vi "FTW-JSON-Object-DeleteElement.vi"(0 "JSON":T1, 5 "Key":string, 11 "error in":errorcluster) -> (4 "JSON out":T1, 6 "Found and Removed?":bool, 15 "error out":errorcluster)   [LabVIEW 2015]
uses:
  core/type/FTW-Type-JSON.ctl
panel:
  # "Inputs"
  # "Outputs"
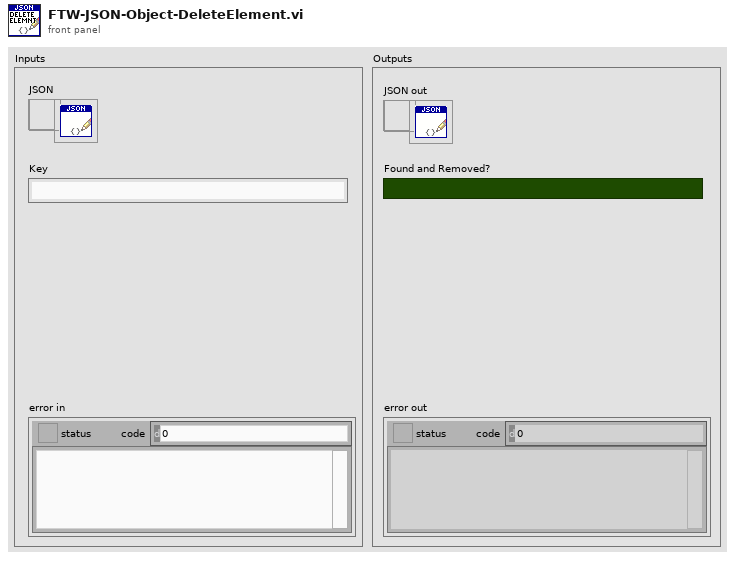
[diagram p1: front panel]
types:
  T1 = typedef "FTW-Type-JSON.ctl" = refnum<data-value>
  T2 = cluster{"FTW-CodeGen-Type":enum16{"FTW-JSON"}, "Object":i64, "EncodingFlags":i64, "DecodingFlags":i64}
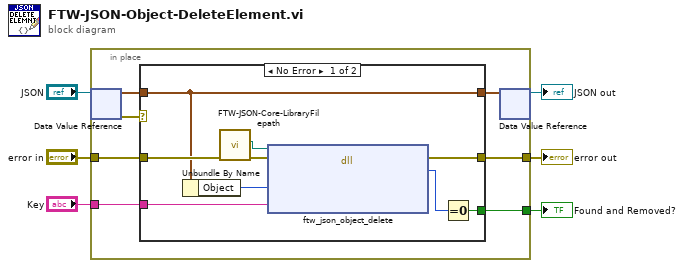
[diagram p0: block diagram]
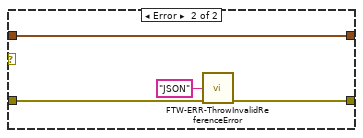
[diagram p2: hidden frame]
diagram:
  n1 = in-place {
    in-place-border: "error in" -> [w9]
    in-place-border: "Key" -> [w13]
    in-place-border: [w12] -> w6
    in-place-border: [w11] -> w1
    n2 = in-place-dvr #1("JSON") -> (w10:T2, w7:errorcluster)
    n3 = case shown="No Error" w7 {
      tunnel: w13 -> [w22 _]
      tunnel: [w21 w23] -> w12
      tunnel: [w19 _] -> w11
      tunnel: w10 -> [w14 w26]
      tunnel: w9 -> [w17 w24]
      tunnel: [w14 w26] -> w8
      frame No Error {
        n4 = Unbundle By Name(w14) -> ("Object"=w18:i64)
        n5 = call "FTW-JSON-Core-LibraryFilepath.vi"("error in"=w17) -> ("error out"=w16:errorcluster, "JSON Library Filepath"=w15:path)  [unwired: 9 in]
        n6 = dll-call lib="?" fn="ftw_json_object_delete"(path in=w15, error in=w16, "JSON Object Pointer"=w18, "Element Key"=w22) -> (error out=w21:errorcluster, "JSON Element Pointer"=w20:i64)  [unwired: 3 in, 1 out]
        n7 = Equal To 0?(x=w20) -> (x = 0?=w19:bool)
      }
      frame Error {
        n8 = call "FTW-ERR-ThrowInvalidReferenceError.vi"("Reference Type"="JSON", "error in"=w24) -> ("error out"=w23:errorcluster)  [unwired: 13 in]
      }
    }
    n9 = in-place-dvr #1(w8) -> (→"JSON out":T1)  [unwired: 1 out]
  }
  "error out" <- w6
  "Found and Removed?" <- w1
